vi "Assert String Not Starts With.vi"(4 "Execution time (s)":dbl=-1.0, 5 "Assert Only? (F)":bool, 6 "error code (1)":i32=1, 7 "Label (\"\")":string, 8 "error in (no error)":errorcluster, 9 "Register with caller test (F)":bool, 10 "Substring":string, 11 "String":string) -> (0 "error out":errorcluster, 2 "Properties.Assert":refnum<class "Properties.Assert.lvclass">)   [LabVIEW 2013, in "Caraya.lvlib" / "Assert.lvclass"]
doc: "Asserts that a string does not start with a substring."
uses:
  Assert.lvclass
  Properties.Assert/Properties.Assert.lvclass
  Properties/Properties.lvclass
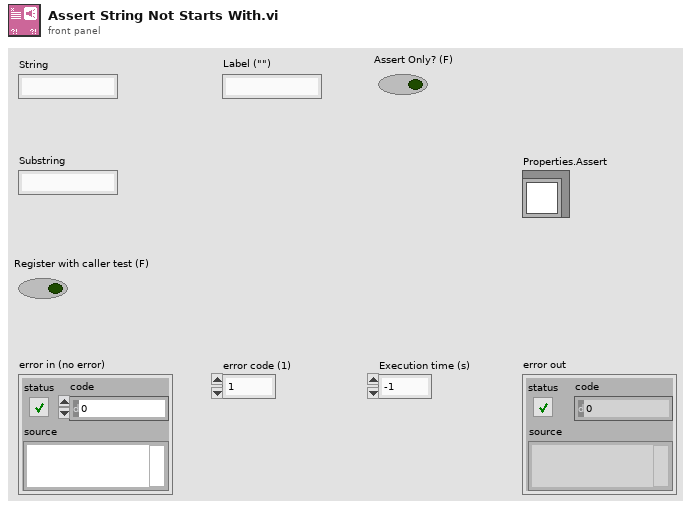
[diagram p1: front panel]
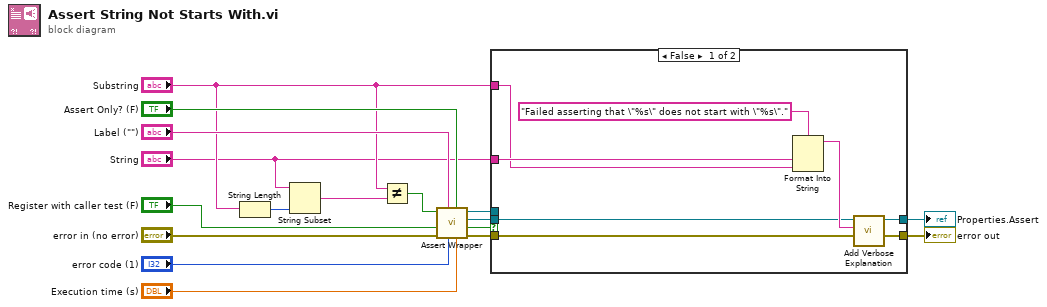
[diagram p0: block diagram]
diagram:
  n1 = String Length(string="Substring") -> (length=w3:i32)
  n2 = String Subset(string="String", length (rest)=w3) -> (substring=w2:string)  [unwired: 1 in]
  n3 = Not Equal?(x="Substring", y=w2) -> (x != y?=w4:bool)
  n4 = call "Assert Wrapper.vi"("Execution time (s)"="Execution time (s)", "Assert Only? (F)"="Assert Only? (F)", "error code (1)"="error code (1)", "Label"="Label (\"\")", "error in (no error)"="error in (no error)", "Register with caller test (F)"="Register with caller test (F)", "Assert?"=w4) -> ("error out"=w7:errorcluster, "Verbose"=w11:bool, "Properties.Assert"=w9:refnum<class "Properties.Assert.lvclass">, "Assert out"=w10:refnum<class "Assert.lvclass">)  [unwired: 1 in]
  n5 = case shown="False" w11 {
    tunnel: w10 -> [_ _]
    tunnel: w9 -> [w20 w27]
    tunnel: [w22 w26] -> w8
    tunnel: w7 -> [w23 w26]
    tunnel: "Substring" -> [w24 _]
    tunnel: "String" -> [w25 _]
    tunnel: [w19 w27] -> w6
    frame False {
      n6 = Format Into String(format string="Failed asserting that \"%s\" does not start with \"%s\".", w25, w24) -> (resulting string=w21:string)  [unwired: 2 in, 1 out]
      n7 = call "Add Verbose Explanation.vi"("error in (no error)"=w23, "Verbose Explanation"=w21, "Properties"=w20) -> ("error out"=w22:errorcluster, "Properties"=w19:refnum<class "Properties.Assert.lvclass">)  [unwired: 7 in]
    }
    frame True {
    }
  }
  "error out" <- w8
  "Properties.Assert" <- w6
